vi "TEB EventFrag= Message.vi"(0 "Event Fragment(s)":string[][](array[string]), 1 "Event Number":i32) -> ()   [LabVIEW 2010]
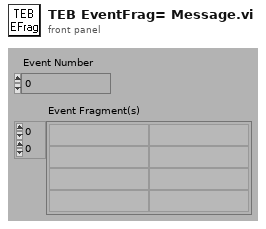
[diagram p1: front panel]
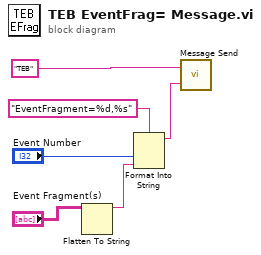
[diagram p0: block diagram]
diagram:
  n1 = Flatten To String(anything="Event Fragment(s)") -> (data string=w2:string)  [unwired: 3 in, 2 out]
  n2 = Format Into String(format string="EventFragment=%d,%s", "Event Number", w2) -> (resulting string=w5:string)  [unwired: 2 in, 1 out]
  n3 = call "Message Send.vi"("Message"=w5, "Destination"="TEB" ("Destination(s)")) -> ()
